vi "Read Keys.vi"(8 "error in (no error)":errorcluster) -> (0 "error out":errorcluster, 3 "Config":T1)   [LabVIEW 2017, in "csm-ini-variable-addon.lvclass"]
uses:
  csm-ini-variable-addon.lvclass
  INI-Static-Variable-Support/LabVIEW-Config/LabVIEW-Config.lvclass
  INI-Static-Variable-Support/LabVIEW-Config/Read Key (DBL).vi
  INI-Static-Variable-Support/LabVIEW-Config/Read Key (Boolean).vi
  INI-Static-Variable-Support/LabVIEW-Config/Read Key (Raw).vi
  INI-Static-Variable-Support/LabVIEW-Config/Read Key (U32).vi
  INI-Static-Variable-Support/LabVIEW-Config/Read Key (String).vi
  INI-Static-Variable-Support/LabVIEW-Config/Read Key (I32).vi
panel:
  out "Key Names":string[](array[string])
  out "Section Names":string[](array[string])
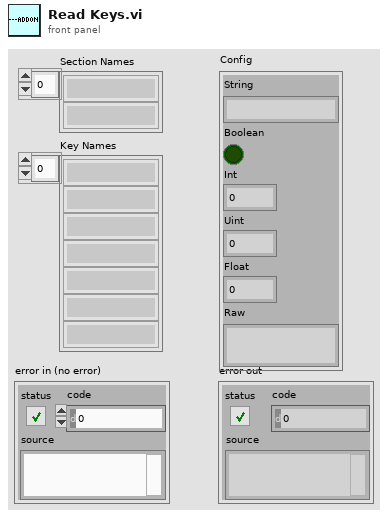
[diagram p1: front panel]
types:
  T1 = cluster{"String":string, "Boolean":bool, "Int":i32, "Uint":u32, "Float":dbl, "Raw":string}
  T2 = typedef "LabVIEW-Config.lvlib/LabVIEW-Config.lvclass/Config.ctl" = cluster{"Path":path, "Lines":string[], "Tokens":T3[], "Modified?":bool, "Cache":cluster{"Valid?":bool, "Key Information":T4[]}}
  T3 = typedef "LabVIEW-Config.lvlib/LabVIEW-Config.lvclass/LineToken.ctl" = enum8{"comment", "section", "key", "more"}
  T4 = typedef "LabVIEW-Config.lvlib/LabVIEW-Config.lvclass/KeyInfo.ctl" = cluster{"Key Indexes":cluster{"Indexes":i32[]}[], "Session Found?":bool, "Key found?":bool, "Session Index":i32}
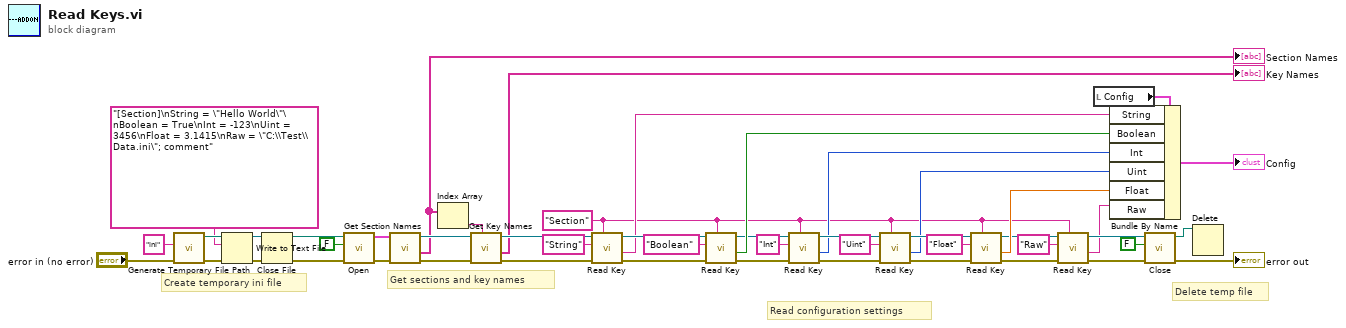
[diagram p0: block diagram]
diagram:
  w3 = "Section" ("Section Name")
  # "Get sections and key names"
  # "Delete temp file"
  # "Read configuration settings"
  # "Create temporary ini file"
  n1 = call <vilib>:"Generate Temporary File Path.vi"("error in (no error)"="error in (no error)", "Temporary File Extension (tmp)"="ini") -> ("error out"=w33:errorcluster, "Unique Temporary File Path"=w30:path)  [unwired: 8 in]
  n2 = Write to Text File(file (use dialog)=w30, text="[Section]\nString = \"Hello World\"\nBoolean = True\nInt = -123\nUint = 3456\nFloat = 3.1415\nRaw = \"C:\\Test\\Data.ini\"; comment", error in=w33) -> (refnum out=w29:refnum<file>, error out=w31:errorcluster)  [unwired: 1 in, 1 out]
  n3 = Close File(refnum=w29, error in=w31) -> (path=w10:path, error out=w11:errorcluster)
  n4 = call "Open.vi"("error in (no error)"=w11, "Create if not exists? (T)"=FALSE, "Path"=w10) -> ("error out"=w47:errorcluster, "Config"=w8:T2)  [unwired: 5 in, 2 out]
  n5 = call "Get Section Names.vi"("error in (no error)"=w47, "Config in"=w8) -> ("error out"=w9:errorcluster, "Section Names"=w2:string[], "Config out"=w6:refnum<class "LabVIEW-Config.lvclass">)  [unwired: 7 in]
  "Section Names" <- w2
  n6 = Index Array(array=w2) -> (element=w1:string)  [unwired: 1 in]
  n7 = call "Get Key Names.vi"("Section Name"=w1, "error in (no error)"=w9, "Config in"=w6) -> ("error out"=w7:errorcluster, "Key Names"=→"Key Names":string[], "Config out"=w5:refnum<class "LabVIEW-Config.lvclass">)  [unwired: 5 in, 1 out]
  n8 = call-poly "Read Key.vi"("Section Name"=w3, "error in (no error)"=w7, "Key Name"="String", "Config in"=w5) -> ("error out"=w44:errorcluster, "Value"=w39:string, "Config out"=w43:refnum<class "LabVIEW-Config.lvclass">)  [unwired: 4 in, 1 out]
  n9 = call-poly "Read Key.vi"("Section Name"=w3, "error in (no error)"=w44, "Key Name"="Boolean", "Config in"=w43) -> ("error out"=w42:errorcluster, "Value"=w38:bool, "Config out"=w36:refnum<class "LabVIEW-Config.lvclass">)  [unwired: 4 in, 1 out]
  n10 = call-poly "Read Key.vi"("Section Name"=w3, "error in (no error)"=w42, "Key Name"="Int", "Config in"=w36) -> ("error out"=w37:errorcluster, "Value"=w22:i32, "Config out"=w27:refnum<class "LabVIEW-Config.lvclass">)  [unwired: 4 in, 1 out]
  n11 = call-poly "Read Key.vi"("Section Name"=w3, "error in (no error)"=w37, "Key Name"="Uint", "Config in"=w27) -> ("error out"=w28:errorcluster, "Value"=w21:u32, "Config out"=w24:refnum<class "LabVIEW-Config.lvclass">)  [unwired: 4 in, 1 out]
  n12 = call-poly "Read Key.vi"("Section Name"=w3, "error in (no error)"=w28, "Key Name"="Float", "Config in"=w24) -> ("error out"=w25:errorcluster, "Value"=w20:dbl, "Config out"=w17:refnum<class "LabVIEW-Config.lvclass">)  [unwired: 4 in, 1 out]
  n13 = call-poly "Read Key.vi"("Section Name"=w3, "error in (no error)"=w25, "Key Name"="Raw", "Config in"=w17) -> ("error out"=w18:errorcluster, "Content"=w14:string, "Config out"=w16:refnum<class "LabVIEW-Config.lvclass">)  [unwired: 4 in, 1 out]
  n14 = local read "Config"() -> (w41:T1)
  n15 = Bundle By Name(cluster=w41, "String"=w39, "Boolean"=w38, "Int"=w22, "Uint"=w21, "Float"=w20, "Raw"=w14) -> (→"Config":T1)
  n16 = call "Close.vi"("error in (no error)"=w18, "Write if modified? (T)"=FALSE, "Config"=w16) -> ("error out"=→"error out":errorcluster, "Path"=w13:path)  [unwired: 7 in]
  n17 = Delete(path (use dialog)=w13) -> ()  [unwired: 4 in, 3 out]
